vi "Calculate_RPM.vi"(7 "ElaspedTime":dbl, 8 "PreviousValueR":dbl, 9 "PreviousValueL":dbl, 10 "CurrentValueR":dbl, 11 "CurrentValueL":dbl) -> (2 "R RPM OUT":dbl, 3 "L RPM OUT":dbl)   [LabVIEW 2017]
panel:
  in  "Counts per Rev":dbl
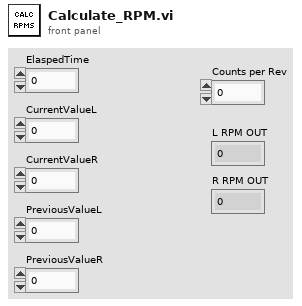
[diagram p1: front panel]
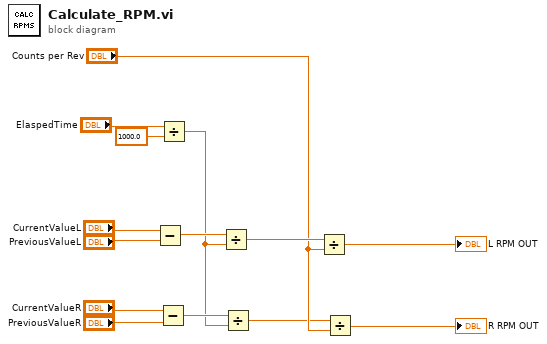
[diagram p0: block diagram]
diagram:
  n1 = Subtract(x="CurrentValueL", y="PreviousValueL") -> (x-y=w10:dbl)
  n2 = Subtract(x="CurrentValueR", y="PreviousValueR") -> (x-y=w9:dbl)
  n3 = Divide(x="ElaspedTime", y=1000.0) -> (x/y=w5:dbl)
  n4 = Divide(x=w10, y=w5) -> (x/y=w8:dbl)
  n5 = Divide(x=w9, y=w5) -> (x/y=w6:dbl)
  n6 = Divide(x=w8, y="Counts per Rev") -> (x/y=→"L RPM OUT":dbl)
  n7 = Divide(x=w6, y="Counts per Rev") -> (x/y=→"R RPM OUT":dbl)
